vi "Movement Control System.vi"(0 "Corner Distances":dbl[](array[numeric])) -> (1 "Left Side PWM":dbl, 2 "Right Side PWM":dbl)   [LabVIEW 2015]
uses:
  Computer_VIs/Localization Mockup.lvlib
panel:
  out "Robot Length":dbl
  out "Robot Width":dbl
  out "Corner Dist 4":dbl
  out "Corner Dist 3":dbl
  out "Corner Dist 2":dbl
  out "Corner Dist 1":dbl
  in  "Dest Y":dbl
  in  "Dest X":dbl
  in  "Start Y":dbl
  in  "Start X":dbl
  # "Moves robot between two specified points.\nNo localization data required.\n\nImplements basic motor control."
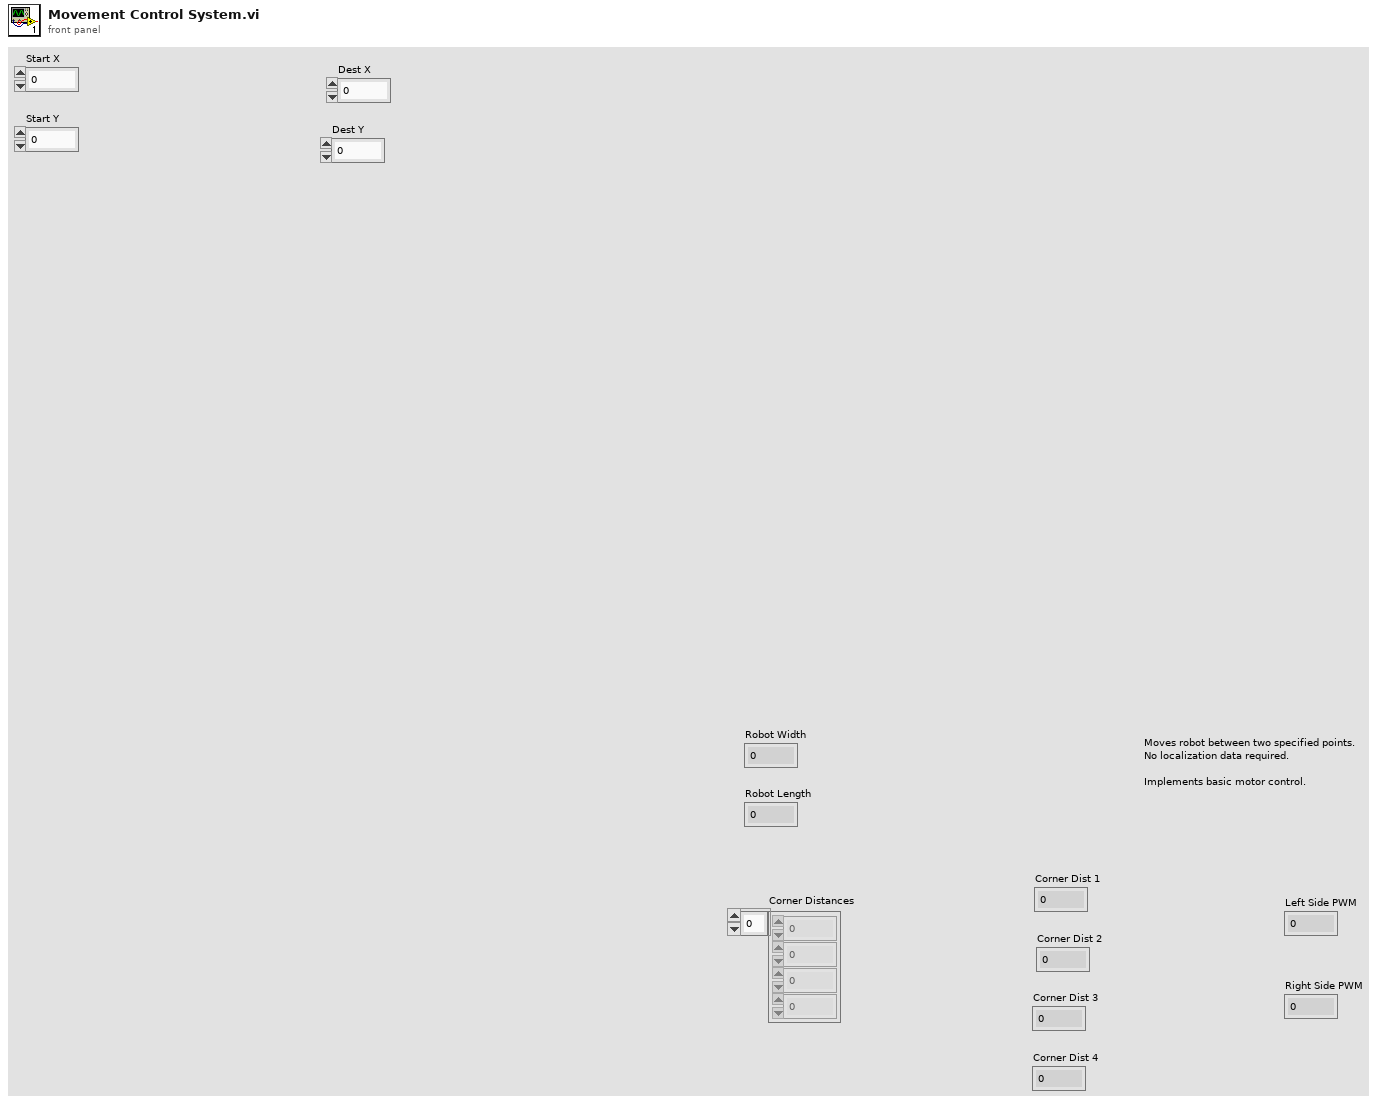
[diagram p1: front panel]
types:
  T1 = cluster{"Corner Distances[0]":dbl, "Corner Distances[1]":dbl, "Corner Distances[2]":dbl, "Corner Distances[3]":dbl, "Corner Distances[4]":dbl, "Corner Distances[5]":dbl, "Corner Distances[6]":dbl, "Corner Distances[7]":dbl, "Corner Distances[8]":dbl}
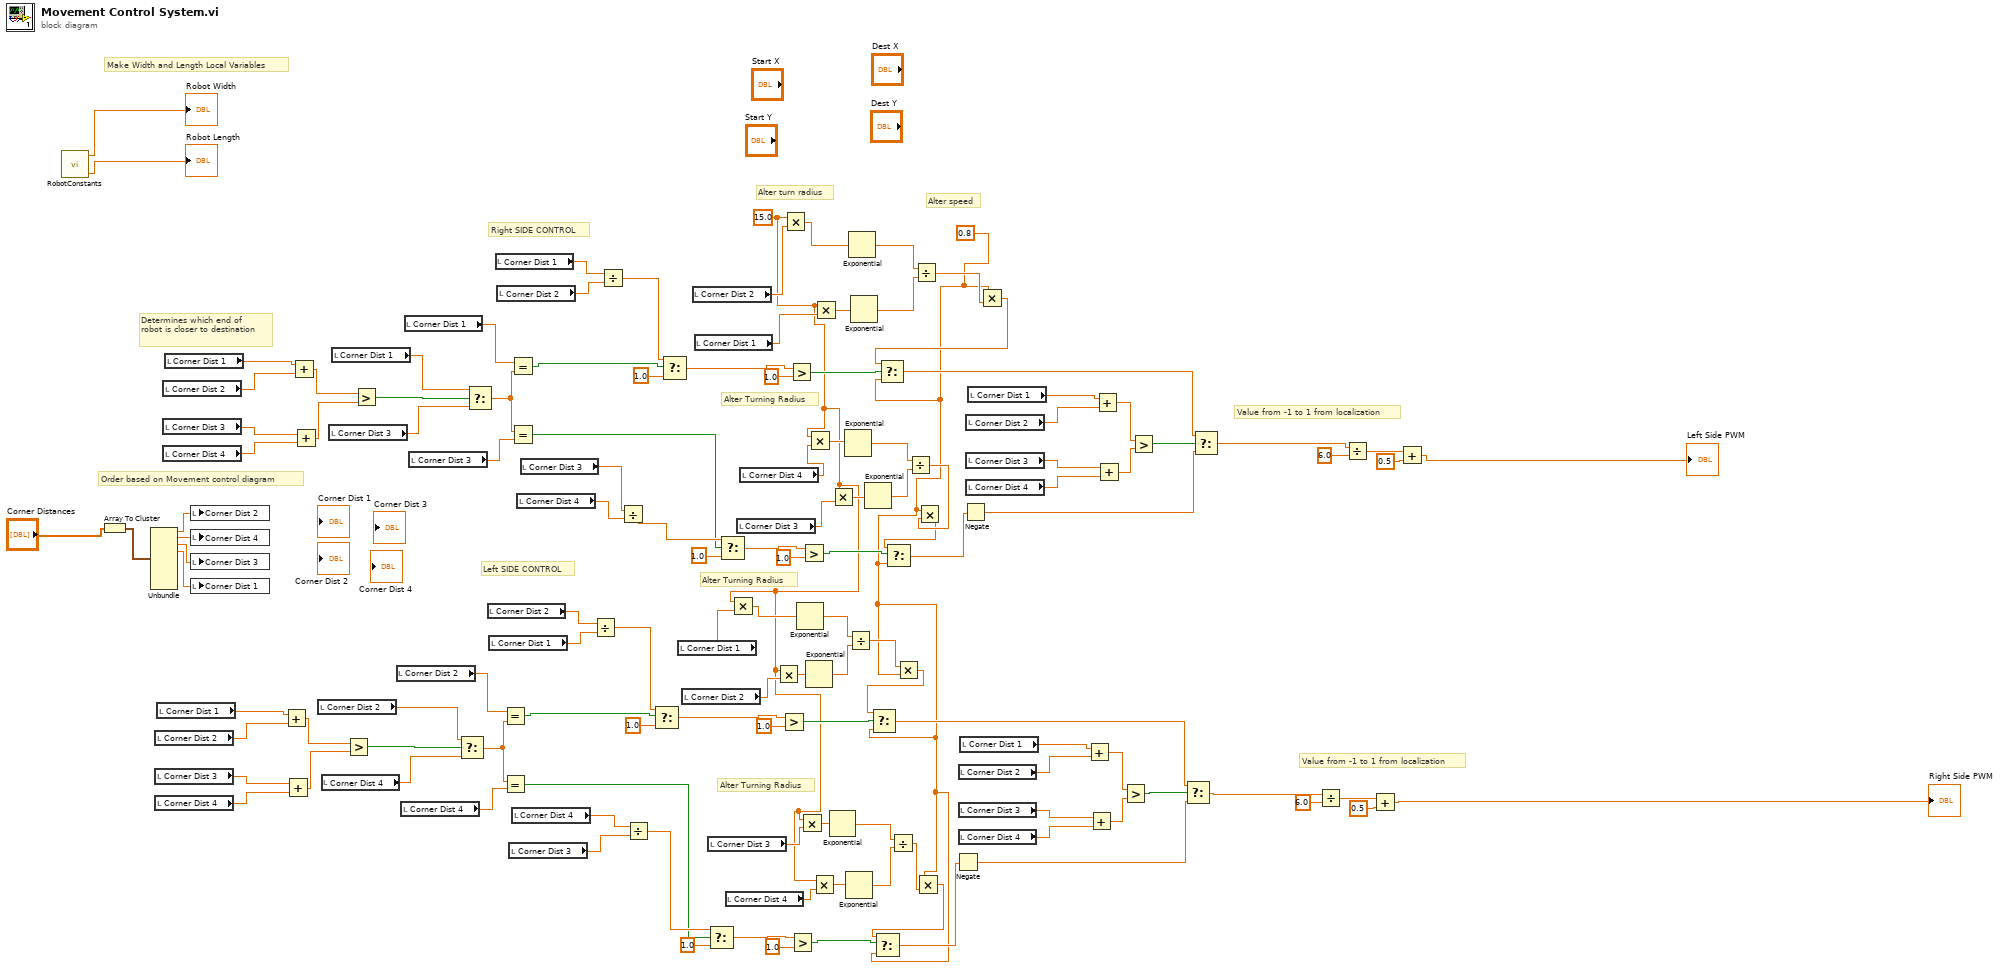
[diagram p0: block diagram]
diagram:
  w2 = 0.8
  w1 = 15.0 ("x")
  # "Alter turn radius"
  # "Make Width and Length Local Variables"
  # "Alter Turning Radius"
  # "Alter Turning Radius"
  # "Alter Turning Radius"
  # "Alter speed"
  # "Value from -1 to 1 from localization"
  # "Order based on Movement control diagram"
  # "Determines which end of \nrobot is closer to destination"
  # "Left SIDE CONTROL"
  # "Right SIDE CONTROL"
  # "Value from -1 to 1 from localization"
  n1 = call "RobotConstants.vi"() -> ("Robot Width (m)"=→"Robot Width":dbl, "Robot Length (m)"=→"Robot Length":dbl)  [unwired: 3 out]
  n2 = Array To Cluster(array="Corner Distances") -> (cluster=w43:T1)
  n3 = Unbundle(w43) -> ("Corner Distances[0]"=w42:dbl, "Corner Distances[1]"=w41:dbl, "Corner Distances[2]"=w40:dbl, "Corner Distances[3]"=w39:dbl)  [unwired: 5 out]
  n4 = local read "Corner Dist 2"() -> (w79:dbl)
  n5 = local read "Corner Dist 3"() -> (w82:dbl)
  n6 = local read "Corner Dist 4"() -> (w81:dbl)
  n7 = local read "Corner Dist 1"() -> (w80:dbl)
  n8 = local read "Corner Dist 2"() -> (w116:dbl)
  n9 = local read "Corner Dist 3"() -> (w119:dbl)
  n10 = local read "Corner Dist 4"() -> (w118:dbl)
  n11 = local read "Corner Dist 1"() -> (w117:dbl)
  n12 = local write "Corner Dist 2"(w42) -> ()
  n13 = local write "Corner Dist 4"(w41) -> ()
  n14 = local write "Corner Dist 3"(w40) -> ()
  n15 = local write "Corner Dist 1"(w39) -> ()
  n16 = Add(x=w80, y=w79) -> (x+y=w85:dbl)
  n17 = Add(x=w82, y=w81) -> (x+y=w84:dbl)
  n18 = Add(x=w117, y=w116) -> (x+y=w122:dbl)
  n19 = Add(x=w119, y=w118) -> (x+y=w121:dbl)
  n20 = local read "Corner Dist 2"() -> (w51:dbl)
  n21 = local read "Corner Dist 4"() -> (w78:dbl)
  n22 = local read "Corner Dist 3"() -> (w115:dbl)
  n23 = local read "Corner Dist 1"() -> (w114:dbl)
  n24 = Greater?(x=w85, y=w84) -> (0:w83:bool)
  n25 = Greater?(x=w122, y=w121) -> (0:w120:bool)
  n26 = local read "Corner Dist 2"() -> (w77:dbl)
  n27 = local read "Corner Dist 4"() -> (w75:dbl)
  n28 = local read "Corner Dist 1"() -> (w113:dbl)
  n29 = local read "Corner Dist 3"() -> (w111:dbl)
  n30 = Select(t=w51, s=w83, f=w78) -> (s? t:f=w76:dbl)
  n31 = Select(t=w114, s=w120, f=w115) -> (s? t:f=w112:dbl)
  n32 = local read "Corner Dist 2"() -> (w45:dbl)
  n33 = local read "Corner Dist 1"() -> (w74:dbl)
  n34 = local read "Corner Dist 1"() -> (w109:dbl)
  n35 = local read "Corner Dist 2"() -> (w110:dbl)
  n36 = Equal?(x=w77, y=w76) -> (x = y?=w73:bool)
  n37 = Equal?(x=w76, y=w75) -> (x = y?=w68:bool)
  n38 = local read "Corner Dist 3"() -> (w70:dbl)
  n39 = Equal?(x=w113, y=w112) -> (x = y?=w108:bool)
  n40 = Equal?(x=w112, y=w111) -> (x = y?=w103:bool)
  n41 = local read "Corner Dist 4"() -> (w71:dbl)
  n42 = local read "Corner Dist 4"() -> (w105:dbl)
  n43 = local read "Corner Dist 3"() -> (w106:dbl)
  n44 = Divide(x=w45, y=w74) -> (x/y=w72:dbl)
  n45 = Divide(x=w109, y=w110) -> (x/y=w107:dbl)
  n46 = Divide(x=w106, y=w105) -> (x/y=w104:dbl)
  n47 = Divide(x=w71, y=w70) -> (x/y=w69:dbl)
  n48 = Select(t=w72, s=w73, f=1.0) -> (s? t:f=w64:dbl)
  n49 = Select(t=w107, s=w108, f=1.0) -> (s? t:f=w99:dbl)
  n50 = local read "Corner Dist 1"() -> (w22:dbl)
  n51 = local read "Corner Dist 2"() -> (w15:dbl)
  n52 = local read "Corner Dist 2"() -> (w26:dbl)
  n53 = local read "Corner Dist 1"() -> (w11:dbl)
  n54 = local read "Corner Dist 3"() -> (w19:dbl)
  n55 = Select(t=w69, s=w68, f=1.0) -> (s? t:f=w67:dbl)
  n56 = Select(t=w104, s=w103, f=1.0) -> (s? t:f=w102:dbl)
  n57 = local read "Corner Dist 4"() -> (w17:dbl)
  n58 = Multiply(x=w1, y=w22) -> (x*y=w21:dbl)
  n59 = local read "Corner Dist 3"() -> (w13:dbl)
  n60 = local read "Corner Dist 4"() -> (w23:dbl)
  n61 = Multiply(x=w1, y=w15) -> (x*y=w16:dbl)
  n62 = Greater?(x=w64, y=1.0) -> (0:w62:bool)
  n63 = Multiply(x=w1, y=w26) -> (x*y=w25:dbl)
  n64 = Greater?(x=w99, y=1.0) -> (0:w97:bool)
  n65 = Greater?(x=w67, y=1.0) -> (0:w65:bool)
  n66 = Exponential(1:w21) -> (0:w29:dbl)
  n67 = Multiply(x=w1, y=w19) -> (x*y=w20:dbl)
  n68 = Greater?(x=w102, y=1.0) -> (0:w100:bool)
  n69 = Exponential(1:w16) -> (0:w30:dbl)
  n70 = Multiply(x=w1, y=w23) -> (x*y=w24:dbl)
  n71 = Multiply(x=w1, y=w17) -> (x*y=w18:dbl)
  n72 = Multiply(x=w1, y=w11) -> (x*y=w12:dbl)
  n73 = Exponential(1:w20) -> (0:w28:dbl)
  n74 = Multiply(x=w1, y=w13) -> (x*y=w14:dbl)
  n75 = Exponential(1:w24) -> (0:w32:dbl)
  n76 = Exponential(1:w18) -> (0:w27:dbl)
  n77 = Divide(x=w29, y=w30) -> (x/y=w6:dbl)
  n78 = Exponential(1:w25) -> (0:w34:dbl)
  n79 = Exponential(1:w12) -> (0:w33:dbl)
  n80 = Exponential(1:w14) -> (0:w31:dbl)
  n81 = Divide(x=w28, y=w27) -> (x/y=w4:dbl)
  n82 = Multiply(x=w6, y=w2) -> (x*y=w5:dbl)
  n83 = Select(t=w5, s=w62, f=w2) -> (s? t:f=w55:dbl)
  n84 = Divide(x=w32, y=w31) -> (x/y=w8:dbl)
  n85 = Divide(x=w34, y=w33) -> (x/y=w10:dbl)
  n86 = Multiply(x=w2, y=w4) -> (x*y=w3:dbl)
  n87 = Select(t=w3, s=w65, f=w2) -> (s? t:f=w53:dbl)
  n88 = Multiply(x=w2, y=w8) -> (x*y=w7:dbl)
  n89 = Select(t=w7, s=w100, f=w2) -> (s? t:f=w87:dbl)
  n90 = Negate(x=w53) -> (-x=w52:dbl)
  n91 = local read "Corner Dist 2"() -> (w58:dbl)
  n92 = local read "Corner Dist 3"() -> (w61:dbl)
  n93 = local read "Corner Dist 4"() -> (w60:dbl)
  n94 = local read "Corner Dist 1"() -> (w59:dbl)
  n95 = Negate(x=w87) -> (-x=w86:dbl)
  n96 = local read "Corner Dist 2"() -> (w93:dbl)
  n97 = local read "Corner Dist 3"() -> (w96:dbl)
  n98 = local read "Corner Dist 4"() -> (w95:dbl)
  n99 = local read "Corner Dist 1"() -> (w94:dbl)
  n100 = Multiply(x=w2, y=w10) -> (x*y=w9:dbl)
  n101 = Select(t=w9, s=w97, f=w2) -> (s? t:f=w90:dbl)
  n102 = Add(x=w59, y=w58) -> (x+y=w57:dbl)
  n103 = Add(x=w61, y=w60) -> (x+y=w56:dbl)
  n104 = Add(x=w94, y=w93) -> (x+y=w92:dbl)
  n105 = Add(x=w96, y=w95) -> (x+y=w91:dbl)
  n106 = Greater?(x=w57, y=w56) -> (0:w54:bool)
  n107 = Greater?(x=w92, y=w91) -> (0:w89:bool)
  n108 = Select(t=w55, s=w54, f=w52) -> (s? t:f=w50:dbl)
  n109 = Select(t=w90, s=w89, f=w86) -> (s? t:f=w88:dbl)
  n110 = Divide(x=w50, y=6.0) -> (x/y=w127:dbl)
  n111 = Divide(x=w88, y=6.0) -> (x/y=w124:dbl)
  n112 = Add(x=w127, y=0.5) -> (x+y=→"Right Side PWM":dbl)
  n113 = Add(x=w124, y=0.5) -> (x+y=→"Left Side PWM":dbl)
